vi "Delacor_lib_QMH_Dequeue Message.vi"(8 "error in":errorcluster, 9 "timeout in ms (-1)":i32=-1, 11 "Message Queue in":refnum<class "RQMHMessageQueue.lvclass">) -> (0 "error out":errorcluster, 1 "Message Data":variant, 2 "Message":string, 3 "Message Queue out":refnum<class "RQMHMessageQueue.lvclass">)   [LabVIEW 2024, in "RQMHMessageQueue.lvclass"]
doc: "This VI pulls messages off the Message Queue.\n____\nDQMH Framework: Palette 7.1.0.1503\nCopyright (c) 2025, DQMH Consortium"
uses:
  RQMHMessageQueue.lvclass
  RQMHMessageQueue.lvclass/RQMHMessageQueue.ctl
  Delacor_lib_QMH_Get Message Queue.vi
  Delacor_lib_QMH_Set Error Debug.vi
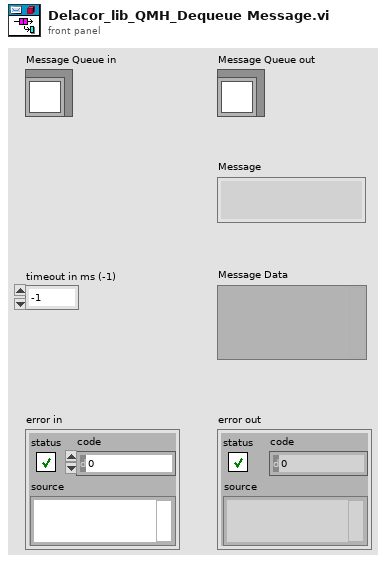
[diagram p1: front panel]
types:
  T1 = typedef "RQMHMessageQueue.lvclass/Delacor_lib_QMH_Message--cluster.ctl" = cluster{"Message":string, "Message Data":variant}
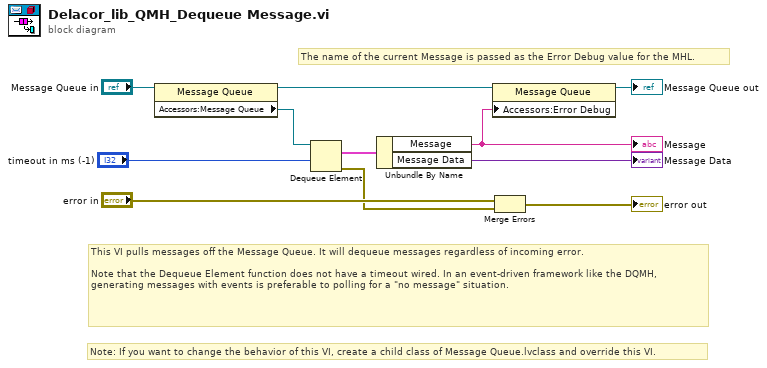
[diagram p0: block diagram]
diagram:
  # "The name of the current Message is passed as the Error Debug value for the MHL."
  # "Note: If you want to change the behavior of this VI, create a child class of Message Queue.lvclass and override this VI."
  # "This VI pulls messages off the Message Queue. It will dequeue messages regardless of incoming error.\n\nNote that the Dequeue Element function does not have a timeout wired. In an event-driven framework like the DQMH, generating messages with events is preferable to polling for a \"no message\" situation."
  n1 = property class="Message Queue"(reference="Message Queue in") -> (reference out=w5:refnum<class "RQMHMessageQueue.lvclass">, "Accessors:Message Queue"=w4:refnum<queue>)  [unwired: 1 in, 1 out]
  n2 = Dequeue Element(queue=w4, timeout in ms (-1)="timeout in ms (-1)") -> (element=w6:T1, error out=w9:errorcluster)  [unwired: 1 in, 2 out]
  n3 = Unbundle By Name(w6) -> ("Message"=w2:string, "Message Data"=→"Message Data":variant)
  "Message" <- w2
  n4 = property class="Message Queue"(reference=w5, "Accessors:Error Debug"=w2) -> (reference out=→"Message Queue out":refnum<class "RQMHMessageQueue.lvclass">)  [unwired: 1 in, 1 out]
  n5 = Merge Errors("error in", w9) -> (→"error out":errorcluster)
